vi "Move Z Raster.vi"(2 "Error In":errorcluster, 3 "Initial Direction":bool=TRUE, 4 "Z Number of Steps":string="0", 5 "Reference In":refnum<class "_Controller.lvclass">) -> (0 "Error Out":errorcluster, 1 "Reference Out":refnum<class "_Controller.lvclass">)   [LabVIEW 2020]
doc: "Uni-axial raster scan logic for the Z direction. Moves in one direction, stopping to account for each scanning point. Once this has been completed (including any remainder steps), the motor performs the same number of total steps but in the opposite direction without stopping.\n\nArgs:\n\nReference In: Incoming communication (reference) between LabView and the scanning rig controller\nZ Number of Steps: Total number of steps to move along that axis\nInitial Direction: Initial direction for the scan\nError In: Checks for any errors with the incoming communication (reference)\n\nReturns:\n\nReference Out: Output communnication (reference) between LabView and controller\nError Out: Checks for any error with output communication (reference)"
uses:
  <instrlib>/Arcus Ethernet Driver 1.0.0/ArcusEthernetComm/classes/Controller/_Controller.lvclass
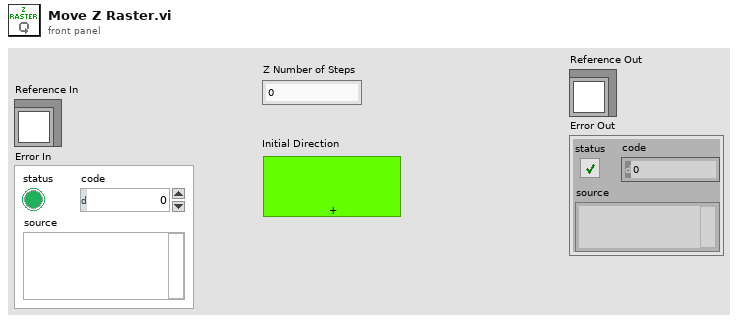
[diagram p1: front panel]
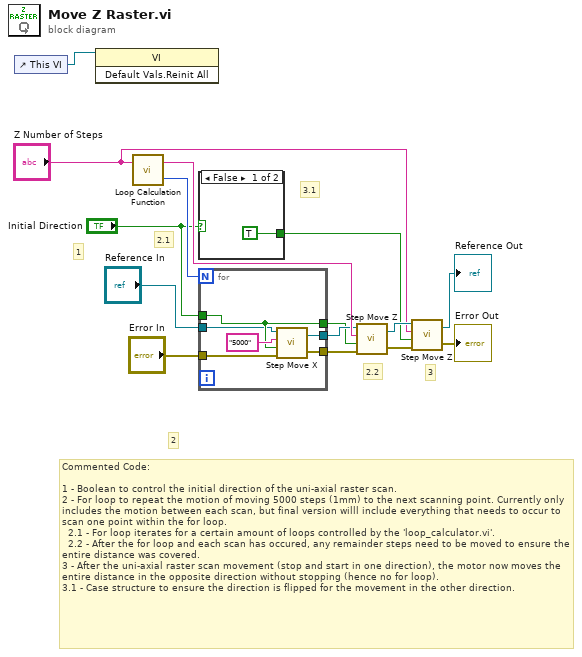
[diagram p0: block diagram]
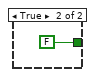
[diagram p2: hidden frame]
diagram:
  # "Commented Code:\n\n1 - Boolean to control the initial direction of the uni-axial raster scan.\n2 - For loop to repeat the motion of moving 5000 steps (1mm) to the next scanning point. Currently only includes the motion between each scan, but final version willl include everything that needs to occur to scan one point within the for loop.\n  2.1 - For loop iterates for a certain amount of loops controlled by the 'loop_calculator.vi'.\n  2.2 - After the for loop and each scan has occured, any remainder steps need to be moved to ensure the entire distance was covered.\n3 - After the uni-axial raster scan movement (stop and start in one direction), the motor now moves the entire distance in the opposite direction without stopping (hence no for loop).\n3.1 - Case structure to ensure the direction is flipped for the movement in the other direction."
  # "2.1"
  # "3.1"
  # "3"
  # "2.2"
  # "1"
  # "2"
  n1 = control-ref of="This VI"() -> (w1:refnum<vi>)
  n2 = invoke class="VI" method="Default Vals.Reinit All"(reference=w1) -> ()  [unwired: 2 in, 3 out]
  n3 = call "Loop Calculation Function.vi"("Number of Steps"="Z Number of Steps") -> ("No. of Scan Points"=w14:i32, "Remainder"=w15:string)  [unwired: 1 in]
  n4 = case shown="False" "Initial Direction" {
    tunnel: [TRUE FALSE] -> w7
    frame False {
    }
    frame True {
    }
  }
  n5 = for {
    N: w14 -> [_]
    tunnel: [w22] -> w12
    tunnel: "Initial Direction" -> [w20]
    tunnel: [w21] -> w11
    tunnel: [w20] -> w10
    tunnel: "Reference In" -> [w19]
    tunnel: "Error In" -> [w18]
    n6 = call "Step Move X.vi"("Error In"=w18, "Direction"=w20, "No. of X Steps"="5000" ("X Steps"), "Reference In"=w19) -> ("Error Out"=w21:errorcluster, "Reference Out"=w22:refnum<class "_Controller.lvclass">)
  }
  n7 = call "Step Move Z.vi"("Error In"=w11, "Direction"=w10, "No. of Z Steps"=w15, "Reference In"=w12) -> ("Error Out"=w8:errorcluster, "Reference Out"=w9:refnum<class "_Controller.lvclass">)
  n8 = call "Step Move Z.vi"("Error In"=w8, "Direction"=w7, "No. of Z Steps"="Z Number of Steps", "Reference In"=w9) -> ("Error Out"=→"Error Out":errorcluster, "Reference Out"=→"Reference Out":refnum<class "_Controller.lvclass">)
